vi "get map range to cluster.vi"(8 "error in (no error)":errorcluster, 11 "data array":string[](array[string])) -> (0 "error IO":errorcluster, 3 "map range":cluster{dbl, dbl, dbl, dbl})   [LabVIEW 2019]
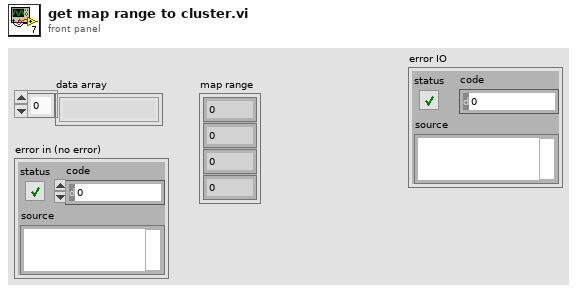
[diagram p1: front panel]
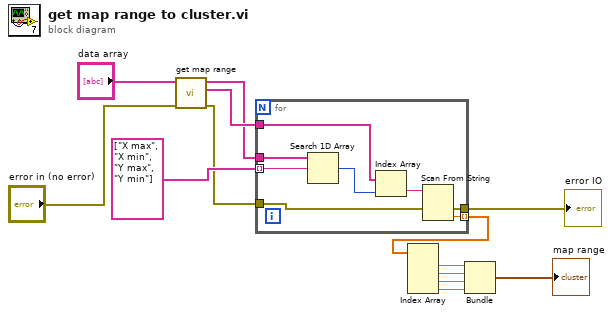
[diagram p0: block diagram]
diagram:
  n1 = call "get map range.vi"("error in (no error)"="error in (no error)", "data array"="data array") -> ("error out"=w2:errorcluster, "<JSON>"=w7:string[], "Item Names"=w5:string[])  [unwired: 7 in]
  n2 = for {
    tunnel: w5 -> [w21]
    tunnel: string[] ["X max", "X min", "Y max", "Y min"] ("Item Names") -> [w20] mode=indexing
    tunnel: w7 -> [w19]
    tunnel: [w16] -> w8 mode=indexing
    tunnel: w2 -> [w15]
    tunnel: [w14] -> w1
    n3 = Search 1D Array(1D array=w21, element=w20) -> (index of element=w18:i32)  [unwired: 1 in]
    n4 = Index Array(array=w19, index=w18) -> (element=w17:string)
    n5 = Scan From String(input string=w17, error in=w15) -> (error out=w14:errorcluster, output 1=w16:dbl)  [unwired: 3 in, 2 out]
  }
  "error IO" <- w1
  n6 = Index Array(array=w8) -> (element #1=w9:dbl, element #2=w10:dbl, element #3=w11:dbl, element #4=w12:dbl)  [unwired: 4 in]
  n7 = Bundle(w9, w10, w11, w12) -> (→"map range":cluster{dbl, dbl, dbl, dbl})  [unwired: 1 in]
